vi "2_32_Fxp_addation.vi"(1 "y":fxp<+/-,32,2>, 2 "x":fxp<+/-,32,2>) -> (0 "x+y":fxp<+/-,33,3> format="%.41g")   [LabVIEW 2020]
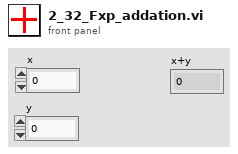
[diagram p1: front panel]
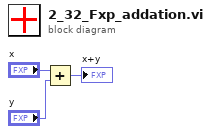
[diagram p0: block diagram]
diagram:
  n1 = Add(x="x", y="y") -> (x+y=→"x+y":fxp<+/-,33,3>)
